vi "RRTWrapper.vi"(8 "error in (no error)":errorcluster, 10 "DLL Path":path, 11 "Input":T2={"seed"=500000, "pathsize"=0, "probGoal"=0.1, "probWaypoint"=0.6, "step"=10.0, "threshold"=10.0, "field_length"=9000.0, "field_width"=6000.0, "startAndEnd"=[[0.0, 0.0], [0.0, 0.0]], "obsList"=[[0.0, 0.0]], "obsLen"=1, "lastTree"=[[0.0, 0.0]], "lastTreeLen"=1, "newTree"=[0.0, 0.0, 0.0, 0.0], "useSimplePath"=0, "debug"=0.0}) -> (0 "error out":errorcluster, 3 "Output":T1)   [LabVIEW 2024]
uses:
  RRTInput.ctl
  RRTOutput.ctl
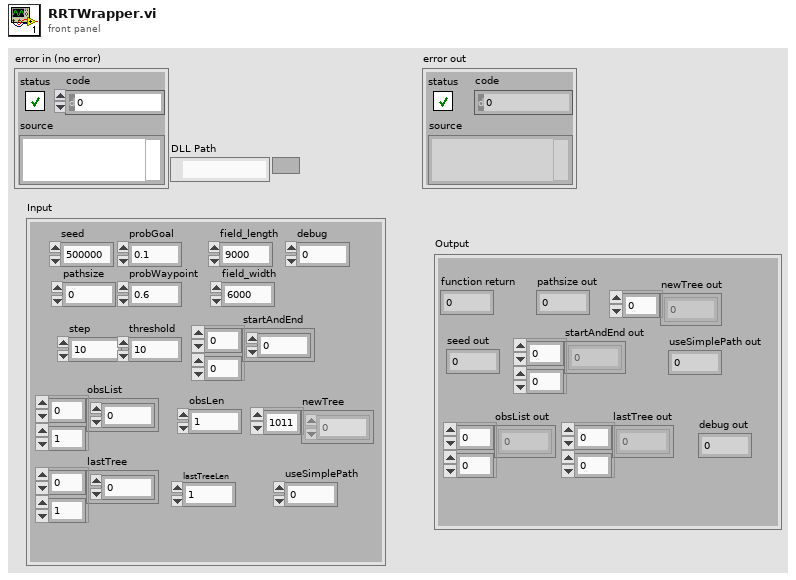
[diagram p1: front panel]
types:
  T1 = typedef "RRTOutput.ctl" = cluster{"function return":i32, "seed out":i32, "pathsize out":i32, "startAndEnd out":sgl[][], "obsList out":sgl[][], "lastTree out":sgl[][], "newTree out":sgl[], "useSimplePath out":i32, "debug out":sgl}
  T2 = typedef "RRTInput.ctl" = cluster{"seed":i32, "pathsize":i32, "probGoal":sgl, "probWaypoint":sgl, "step":sgl, "threshold":sgl, "field_length":sgl, "field_width":sgl, "startAndEnd":sgl[][], "obsList":sgl[][], "obsLen":i32, "lastTree":sgl[][], "lastTreeLen":i32, "newTree":sgl[], "useSimplePath":i32, "debug":sgl}
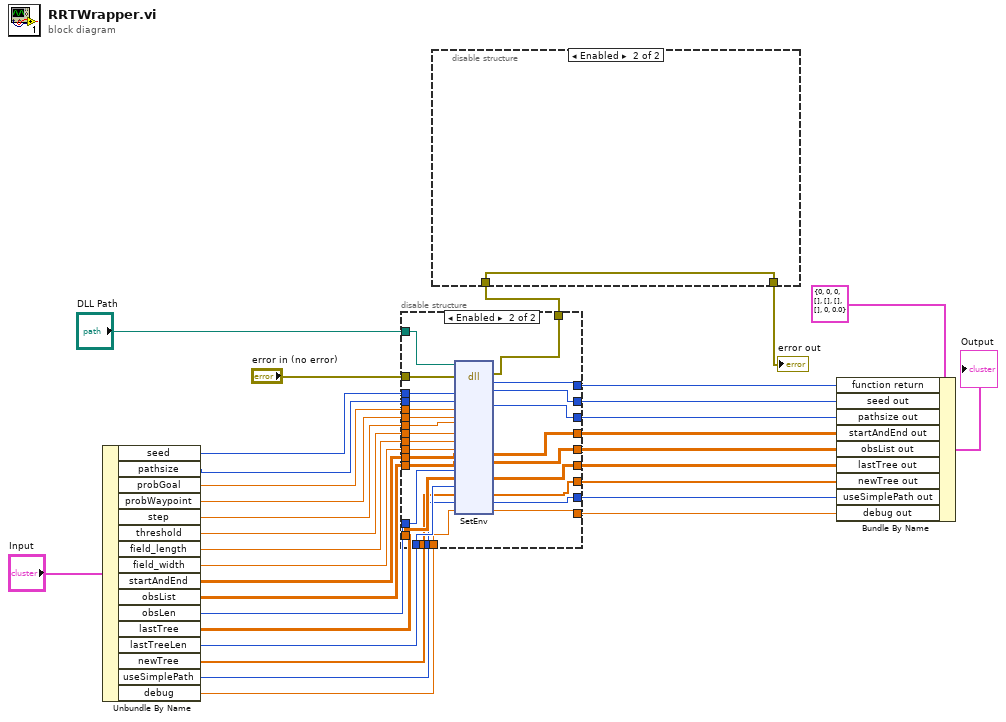
[diagram p0: block diagram]
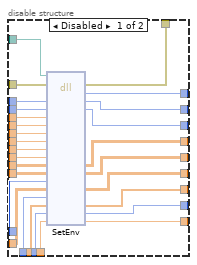
[diagram p2: hidden frame]
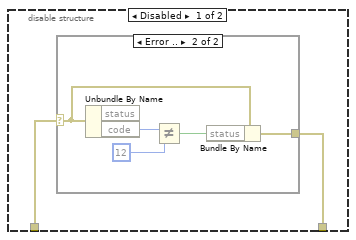
[diagram p3: hidden frame]
diagram:
  n1 = Unbundle By Name("Input") -> ("seed"=w28:i32, "pathsize"=w27:i32, "probGoal"=w26:sgl, "probWaypoint"=w25:sgl, "step"=w24:sgl, "threshold"=w23:sgl, "field_length"=w22:sgl, "field_width"=w21:sgl, "startAndEnd"=w20:sgl[][], "obsList"=w19:sgl[][], "obsLen"=w18:i32, "lastTree"=w17:sgl[][], "lastTreeLen"=w16:i32, "newTree"=w15:sgl[], "useSimplePath"=w14:i32, "debug"=w13:sgl)
  n2 = disable-structure shown="Enabled" {
    disable-tunnel: "error in (no error)" -> [w60 w87]
    disable-tunnel: w28 -> [w59 w86]
    disable-tunnel: w27 -> [w58 w85]
    disable-tunnel: w26 -> [w57 w84]
    disable-tunnel: w25 -> [w56 w83]
    disable-tunnel: w24 -> [w55 w82]
    disable-tunnel: w23 -> [w54 w81]
    disable-tunnel: w22 -> [w53 w80]
    disable-tunnel: w21 -> [w52 w79]
    disable-tunnel: w20 -> [w51 w78]
    disable-tunnel: w19 -> [w50 w77]
    disable-tunnel: w18 -> [w49 w76]
    disable-tunnel: w17 -> [w48 w75]
    disable-tunnel: w16 -> [w47 w74]
    disable-tunnel: w15 -> [w46 w73]
    disable-tunnel: w14 -> [w45 w72]
    disable-tunnel: w13 -> [w44 w71]
    disable-tunnel: [w43 w62] -> w12
    disable-tunnel: [w42 w63] -> w11
    disable-tunnel: [w41 w64] -> w10
    disable-tunnel: [w40 w65] -> w9
    disable-tunnel: [w39 w66] -> w8
    disable-tunnel: [w38 w67] -> w7
    disable-tunnel: [w37 w68] -> w6
    disable-tunnel: [w36 w69] -> w5
    disable-tunnel: [w35 w70] -> w4
    disable-tunnel: "DLL Path" -> [w34 w88]
    disable-tunnel: [w33 w61] -> w2
    frame Disabled {
      n3 = dll-call lib="C:/Users/ebert/Documents/codes/SSL/repo/SSL_AI/RRT/DLL-RRT/x64/RRT.*" fn="SetEnv"(path in=w34, error in=w60, "seed"=w59, "pathsize"=w58, "probGoal"=w57, "probWaypoint"=w56, "step"=w55, "threshold"=w54, "field_length"=w53, "field_width"=w52, "startAndEnd"=w51, "obsList"=w50, "obsLen"=w49, "lastTree"=w48, "lastTreeLen"=w47, "newTree"=w46, "useSimplePath"=w45, "debug"=w44) -> (error out=w33:errorcluster, "return type"=w43:i32, "seed"=w42:i32, "pathsize"=w41:i32, "startAndEnd"=w40:sgl[][], "obsList"=w39:sgl[][], "lastTree"=w38:sgl[][], "newTree"=w37:sgl[], "useSimplePath"=w36:i32, "debug"=w35:sgl)  [unwired: 9 in, 1 out]
    }
    frame Enabled {
      n4 = dll-call lib="C:/Users/as119/OneDrive/Documentos/roboIME/SSL_AI/RRT/RRT-DLL/x64/RRT.*" fn="SetEnv"(path in=w88, error in=w87, "seed"=w86, "pathsize"=w85, "probGoal"=w84, "probWaypoint"=w83, "step"=w82, "threshold"=w81, "field_length"=w80, "field_width"=w79, "startAndEnd"=w78, "obsList"=w77, "obsLen"=w76, "lastTree"=w75, "lastTreeLen"=w74, "newTree"=w73, "useSimplePath"=w72, "debug"=w71) -> (error out=w61:errorcluster, "return type"=w62:i32, "seed"=w63:i32, "pathsize"=w64:i32, "startAndEnd"=w65:sgl[][], "obsList"=w66:sgl[][], "lastTree"=w67:sgl[][], "newTree"=w68:sgl[], "useSimplePath"=w69:i32, "debug"=w70:sgl)  [unwired: 9 in, 1 out]
    }
  }
  n5 = disable-structure shown="Enabled" {
    disable-tunnel: w2 -> [w90 w97]
    disable-tunnel: [w89 w97] -> w1
    frame Disabled {
      n6 = case shown="Error .." w90 {
        selector: w90 -> [w91 w94]
        tunnel: [w91 w92] -> w89
        frame No Error {
        }
        frame Error {
          n7 = Unbundle By Name(w94) -> ("code"=w96:i32)  [unwired: 1 out]
          n8 = Not Equal?(x=w96, y=12) -> (x != y?=w93:bool)
          n9 = Bundle By Name(cluster=w94, "status"=w93) -> (w92:errorcluster)
        }
      }
    }
    frame Enabled {
    }
  }
  "error out" <- w1
  n10 = Bundle By Name(cluster=T1 {"function return"=0, "seed out"=0, "pathsize out"=0, "startAndEnd out"=[], "obsList out"=[], "lastTree out"=[], "newTree out"=[], "useSimplePath out"=0, "debug out"=0.0} ("Output"), "function return"=w12, "seed out"=w11, "pathsize out"=w10, "startAndEnd out"=w9, "obsList out"=w8, "lastTree out"=w7, "newTree out"=w6, "useSimplePath out"=w5, "debug out"=w4) -> (→"Output":T1)
